vi "contrast move.vi"(8 "error in (no error)":errorcluster, 9 "Position in":T1, 10 "speed":dbl=100.0 format="%#_13g", 11 "Target degree":dbl) -> (0 "error out":errorcluster, 1 "Position out":T1)   [LabVIEW 2019]
uses:
  position cluster.ctl
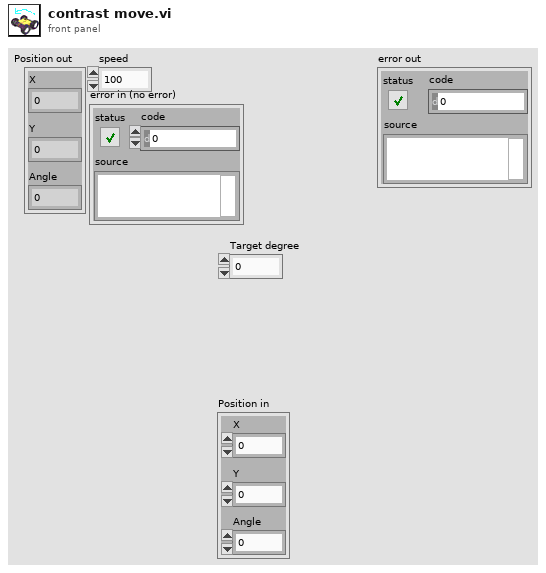
[diagram p1: front panel]
types:
  T1 = typedef "position cluster.ctl" = cluster{"X":dbl, "Y":dbl, "Angle":dbl}
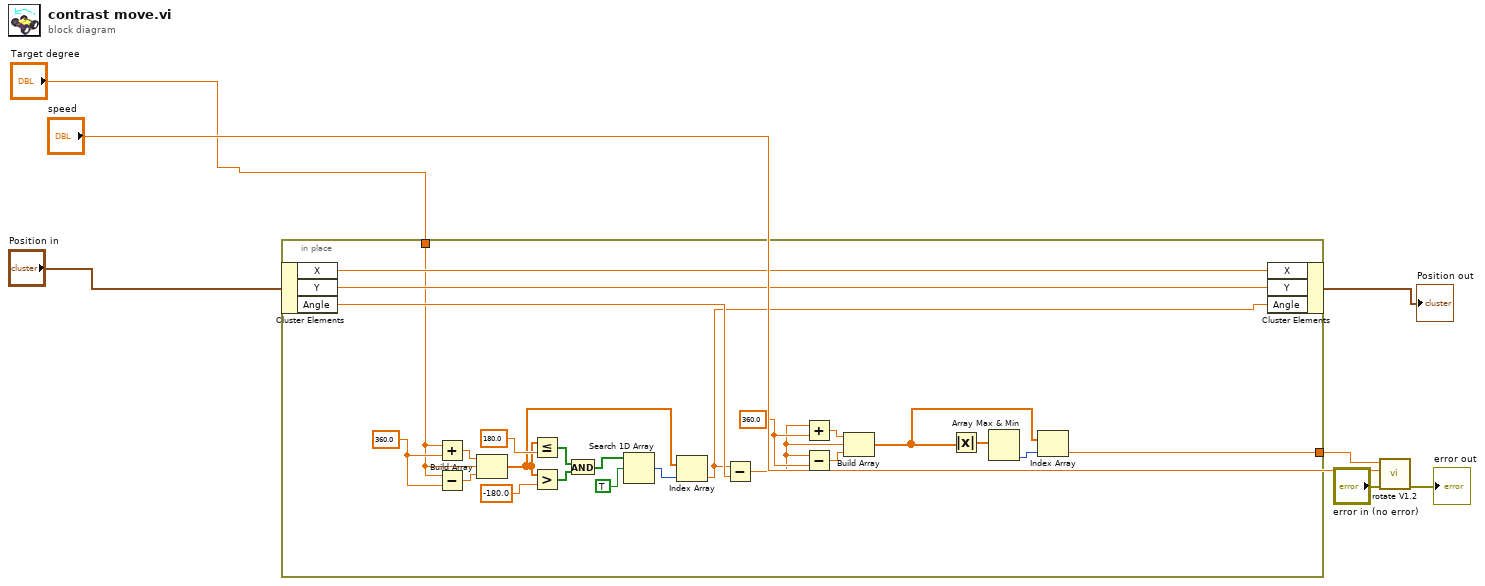
[diagram p0: block diagram]
diagram:
  n1 = in-place {
    in-place-border: "Target degree" -> [w9]
    in-place-border: [w8] -> w5
    w17 = 360.0
    w29 = 360.0
    n2 = in-place-cluster #1("Position in") -> ("X"=w31:dbl, "Y"=w30:dbl, "Angle"=w18:dbl)
    n3 = Add(x=w9, y=w29) -> (x+y=w28:dbl)
    n4 = Subtract(x=w9, y=w29) -> (x-y=w27:dbl)
    n5 = Build Array(w28, w9, w27) -> (w19:dbl[])
    n6 = Less Or Equal?(x=w19, y=180.0) -> (x <= y?=w24:bool[])
    n7 = Greater?(x=w19, y=-180.0) -> (0:w23:bool[])
    n8 = And(x=w24, y=w23) -> (x .and. y?=w22:bool[])
    n9 = Search 1D Array(1D array=w22, element=TRUE) -> (index of element=w20:i32)  [unwired: 1 in]
    n10 = Index Array(array=w19, index=w20) -> (element=w10:dbl)
    n11 = Subtract(x=w10, y=w18) -> (x-y=w15:dbl)
    n12 = Add(x=w15, y=w17) -> (x+y=w16:dbl)
    n13 = Subtract(x=w15, y=w17) -> (x-y=w14:dbl)
    n14 = Build Array(w16, w15, w14) -> (w11:dbl[])
    n15 = Absolute Value(x=w11) -> (abs(x)=w13:dbl[])
    n16 = Array Max & Min(array=w13) -> (min index (indices)=w12:i32)  [unwired: 3 out]
    n17 = Index Array(array=w11, index=w12) -> (element=w8:dbl)
    n18 = in-place-cluster #1("X"=w31, "Y"=w30, "Angle"=w10) -> (→"Position out":T1)
  }
  n19 = call "rotate V1.2.vi"("error in (no error)"="error in (no error)", "speed"="speed", "degree"=w5) -> ("error out"=→"error out":errorcluster)  [unwired: 8 in]
